vi "Ex 06 - B-Scan (DVR).vi"() -> ()   [LabVIEW 2015]
uses:
  <instrlib>/MicroPulse/Public/Data/Datatypes/MP - data formatting.ctl
  <instrlib>/MicroPulse/Public/Data/Datatypes/MP - amplitude reporting mode.ctl
  <instrlib>/MicroPulse/Public/Data/Datatypes/MP - averaging.ctl
  <instrlib>/MicroPulse/Public/Data/Datatypes/MP - transmit parameters.ctl
  <instrlib>/MicroPulse/Public/Data/Datatypes/MP - pulser voltage.ctl
  <instrlib>/MicroPulse/Public/Data/Datatypes/MP - pulse damping.ctl
  <instrlib>/MicroPulse/Public/Data/Datatypes/MP - test parameters.ctl
  <instrlib>/MicroPulse/Public/Data/Datatypes/MP - receive parameters.ctl
  <instrlib>/MicroPulse/Public/Data/Datatypes/MP - display gate.ctl
  <instrlib>/MicroPulse/Public/Data/Datatypes/MP - waveform type.ctl
  <instrlib>/MicroPulse/Public/Data/Datatypes/MP - analogue filter.ctl
  <instrlib>/MicroPulse/Public/Data/Datatypes/MP - frequency filter.ctl
  <instrlib>/MicroPulse/Public/Data/Datatypes/MP - digital filtering.ctl
  <instrlib>/MicroPulse/Public/Data/Datatypes/MP - high pass filter.ctl
  <instrlib>/MicroPulse/Public/Data/Datatypes/MP - low pass filter.ctl
  <instrlib>/MicroPulse/Public/Data/Datatypes/TCP config.ctl
  <instrlib>/MicroPulse/Public/Data/Datatypes/MP - multi-gate inspection.ctl
  <instrlib>/MicroPulse/Public/Data/Datatypes/MP - multigate inspection gate parameters.ctl
  <instrlib>/MicroPulse/Public/Data/Datatypes/MP - hysteresis level.ctl
  <instrlib>/MicroPulse/Public/Data/Datatypes/MP - multigate mode.ctl
  <instrlib>/MicroPulse/Public/Data/Datatypes/MP - echo gate parameters.ctl
  <instrlib>/MicroPulse/Public/Data/Datatypes/MP - echo gate mode.ctl
  <instrlib>/MicroPulse/Public/Data/Datatypes/MP - data output format.ctl
  <instrlib>/MicroPulse/Public/Data/Datatypes/MP - sample frequency.ctl
  <instrlib>/MicroPulse/Public/Data/Datatypes/MP - instrument type.ctl
  <instrlib>/MicroPulse/Public/Data/Datatypes/MP - fly scan range.ctl
  <instrlib>/MicroPulse/Public/Data/Datatypes/MP - inspection direction.ctl
  <instrlib>/MicroPulse/Public/Data/Datatypes/MP - encoder settings.ctl
  <instrlib>/MicroPulse/Public/Data/Datatypes/MP - encoder type.ctl
  <instrlib>/MicroPulse/Public/Data/Datatypes/MP - request system status.ctl
  <instrlib>/MicroPulse/Public/Data/Datatypes/MP - encoder mode.ctl
  <instrlib>/MicroPulse/Public/Data/Datatypes/MP - fly scan range (relative).ctl
  <instrlib>/MicroPulse/Public/Data/Datatypes/MP - inspection direction (relative).ctl
  <instrlib>/MicroPulse/Public/Data/Datatypes/MP - fly scan range (timed).ctl
  <instrlib>/MicroPulse/Public/Data/Datatypes/PNDT - colour map selector.ctl
  <instrlib>/MicroPulse/Examples/SubVIs/Main Program State - Enum.ctl
  <instrlib>/MicroPulse/Public/Data/Datatypes/MP - fly inspection tests.ctl
  <instrlib>/MicroPulse/Public/Helper VIs/Low Level/FGV - B-Scan Active - Action [Enum].ctl
  <vilib>/ErrorRing/Error Ring.xnode
  <instrlib>/MicroPulse/MicroPulse_Driver.lvlib
panel:
  in  "Centre Cursor":bool
  in  "Get Status":bool
  in  "Colour Map":T1
  out "B-Scan In Progress?":bool
  in  "Stop Test":bool
  out "B-Scan Chart":u16[][](graph)
  in  "Request System Status":T2 caption="[STS]"
  out "Current Position":dbl format="%#_6f mm"
  in  "Test Tab":T3(tab)
  in  "Data Formatting":T4={"Amplitude Mode"=enum."Peaks + Ascan for Multigate", "Averaging"=enum."None", "Coupling Level"=0} {"Coupling Level" max=4095 step=1}
  in  "Transmit Parameters":T7={"Pulse Voltage"=enum."50V", "Pulse Shape"={"Damping"=enum."660W", "Width"=250}} {"Pulse Shape"."Width" min=16 max=1010 step=50 format="%.0fns"}
  in  "Test Parameters":T10={"Test No."=1, "Tx Channel"=1, "Rx Channel"=1} {"Rx Channel" min=1 max=1024; "Tx Channel" min=1 max=1024}
  in  "Receive Parameters":T11={"Display Gate"={"Start"=0.0, "Length"=100.0}, "Delay"=0.0, "Waveform Type"=enum."Rectified Signal", "Gain"=50.0, "Analogue Filtering"={"Bandpass"=enum."No change", "Smoothing"=1}, "Digital Filtering"={"High Pass Filter"=enum."None", "Low Pass Filter"=enum."None"}} {"Delay" format="%#_g us"; "Display Gate"."Length" min=0.0 max=64000.0 step=1.0 format="%#_g us"; "Display Gate"."Start" min=0.0 max=64000.0 step=1.0 format="%#_g us"; "Analogue Filtering"."Smoothing" min=1 max=11 step=1; "Gain" min=-6.0 max=70.0 step=0.25 format="%.2fdB"}
  in  "Multi Gate Inspection":T19={"Gate 1"={"Start (us)"=15.0, "Length (us)"=10.0, "Threshold"=80, "Enabled?"=TRUE, "Max # Peaks"=8, "Hysteresis"=enum."6dB", "Mode"=enum."All Peaks In Gate", "Inverted?"=FALSE, "Colour "=16716306}, "Gate 2"={"Start (us)"=30.0, "Length (us)"=10.0, "Threshold"=50, "Enabled?"=TRUE, "Max # Peaks"=8, "Hysteresis"=enum."6dB", "Mode"=enum."All Peaks In Gate", "Inverted?"=FALSE, "Colour "=641024}, "Gate 3"={"Start (us)"=50.0, "Length (us)"=10.0, "Threshold"=30, "Enabled?"=TRUE, "Max # Peaks"=8, "Hysteresis"=enum."6dB", "Mode"=enum."All Peaks In Gate", "Inverted?"=FALSE, "Colour "=4532}, "Gate 4"={"Start (us)"=65.0, "Length (us)"=10.0, "Threshold"=10, "Enabled?"=TRUE, "Max # Peaks"=8, "Hysteresis"=enum."6dB", "Mode"=enum."All Peaks In Gate", "Inverted?"=FALSE, "Colour "=8978537}} {"Gate 4"."Max # Peaks" min=1 max=80 step=1; "Gate 4"."Threshold" min=10 step=10; "Gate 4"."Length (us)" min=0.0 max=96000.0 step=1.0; "Gate 4"."Start (us)" min=0.0 max=64000.0 step=1.0; "Gate 3"."Max # Peaks" min=1 max=80 step=1; "Gate 3"."Threshold" min=10 step=10; "Gate 3"."Length (us)" min=0.0 max=96000.0 step=1.0; "Gate 3"."Start (us)" min=0.0 max=64000.0 step=1.0; "Gate 2"."Max # Peaks" min=1 max=80 step=1; "Gate 2"."Threshold" min=10 step=10; "Gate 2"."Length (us)" min=0.0 max=96000.0 step=1.0; "Gate 2"."Start (us)" min=0.0 max=64000.0 step=1.0; "Gate 1"."Max # Peaks" min=1 max=80 step=1; "Gate 1"."Threshold" min=10 step=10; "Gate 1"."Length (us)" min=0.0 max=96000.0 step=1.0; "Gate 1"."Start (us)" min=0.0 max=64000.0 step=1.0}
  in  "Echo Gate Parameters":T23={"Start (us)"=15.0, "Length (us)"=20.0, "Threshold"=10, "Colour"=2731480} {"Threshold" min=10 max=4095 step=10; "Length (us)" min=0.0 max=96000.0 step=1.0; "Start (us)" min=0.0 max=64000.0 step=1.0}
  in  "Echo Gate Mode":T24
  in  "Encoder Reporting Mode":T25=enum."32-bit + LLC" caption="[ENCM]"
  in  "Set Position":bool
  in  "Position To Set":dbl caption="mm"
  in  "Encoder Settings":T26={"Encoder Type"=enum."Quadrature", "Counts/mm"=100, "Enable Termination?"=FALSE, "Multiplier"=2, "Backlash Period (s)"=10.0, "Encoder Filter"=0} {"Encoder Filter" max=255; "Backlash Period (s)" min=0.0005 max=10.0 step=0.0005; "Multiplier" min=1 max=100000; "Counts/mm" min=1 max=100000}
  in  "Axis No.":u8=1 min=1 max=4
  in  "Scan Choice":T28(tab)
  in  "FLZ Scan definition":T29={"Scan Start"=0.0, "Scan Length"=280.0, "Inspection Resolution"=0.5, "Direction"=enum."Forwards"} {"Inspection Resolution" format="%#_6f"; "Scan Start" format="%#_6f"; "Scan Length" format="%#_6f"}
  in  "Start FLZ Test":bool
  in  "FLR Scan definition":T31={"Scan Length"=0.0, "Inspection Resolution"=1.0, "Direction"=enum."Bidirectional"} {"Inspection Resolution" format="%#_6f"; "Scan Length" format="%#_6f"}
  in  "Start FLR Test":bool
  out "Scan Timer Enabled?":bool
  in  "Start Timed Test":bool
  in  "Timed Scan definition":T33={"Max Scan Length"=0, "Update Rate"=1000, "Direction"=enum."Forwards"} {"Update Rate" format="%#_6f"; "Max Scan Length" format="%#_6f"}
  out "Instrument Type":T34
  out "Sample Frequency out":T35 caption="Sample Frequency"
  out "Stop":bool
  in  "Sample Frequency":T35
  in  "PRF":u16=20000 caption="[PRF]" min=1 max=20000 step=100 format="%dHz"
  in  "Data Output Format":T36=enum."8-bit Mode" caption="[DOF]"
  in  "Gate No.":i32=1
  out "peak data":cluster{"Time":dbl[], "Level":u16[]} {"Time" format="%_6g"}
  out "A-Scan + Peaks":cluster{"timebase":dbl[], "data":u16[]}[](graph) caption="A-Scan + Peaks Test 1"
  in  "Acquire Single Scan":bool
  in  "Stop Acquisition":bool
  in  "Start Acquisition":bool
  out "Command List":string
  in  "QUIT":bool
  out "running average PRF":dbl format="%0.2f"
  out "live error out":errorcluster
  out "message count":i32
  out "System Messages":string
  in  "TCP config":T37={"Connection ID"=refnum, "IP address"="10.1.1.2", "host port"=1067, "OC timeout"=5000, "Read timeout"=2000, "Write timeout"=100} {"Write timeout" format="%dms"; "Read timeout" format="%dms"; "OC timeout" format="%dms"}
  # "Example 06 - B-Scans\n\nSet all controls to the required values\nbefore running the VI.\n\nWhile running, test parameters may NOT be  changed."
  # "Multiplier of 2 sets the inspection resolution to 1/2 of the base unit.\nBase unit is set by  \"Counts/mm\""
  # "Set Current Position"
  # "Set to zero for unlimited points. Requires manual stop."
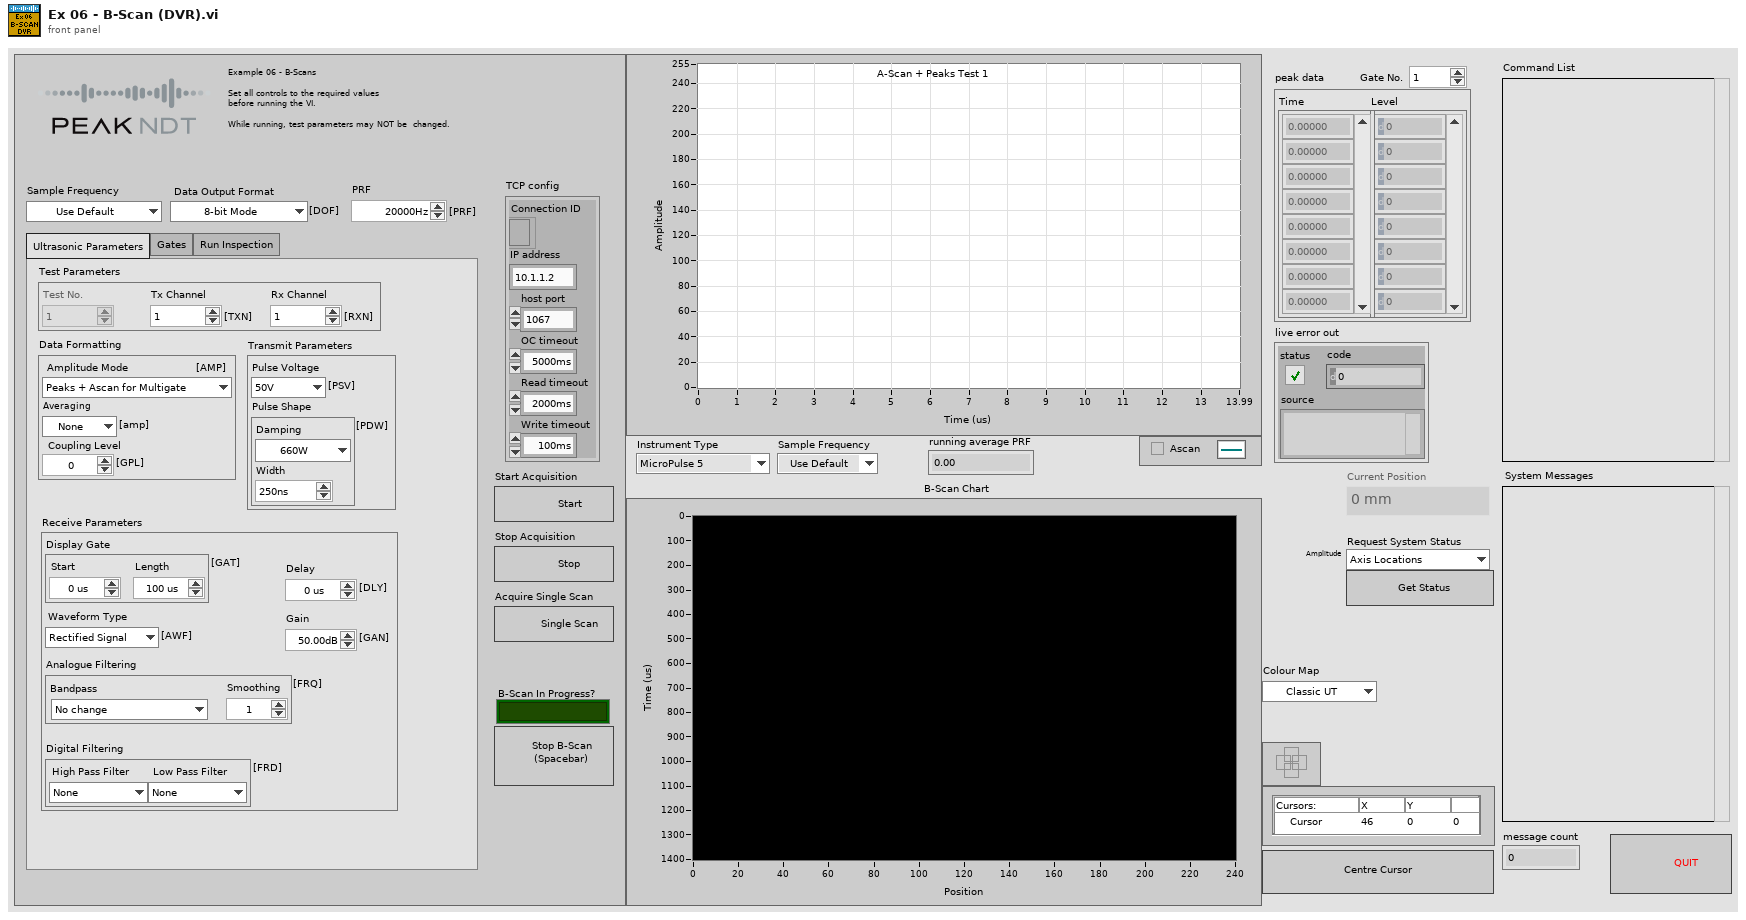
[diagram p1: front panel]
types:
  T1 = typedef "MicroPulse_Driver.lvlib/PNDT - colour map selector.ctl" = enum16{"Classic UT", "Ultrasonic", "Inverse Grey", "Grey Scale", "TOFD", "Fire", "Rainbow", "Ice", "Original"}
  T2 = typedef "MicroPulse_Driver.lvlib/MP - request system status.ctl" = enum16{"Axis Locations", "MPE settings", "BKL settings", "SPA settings", "I/O status", "RST elapsed time", "System Status", "Temperatures", "System Log", "Erase system Log", "RST message", "Master System Msg", "Slave System Msg"}
  T3 = enum32{"Ultrasonic Parameters", "Gates", "Run Inspection"}
  T4 = typedef "MicroPulse_Driver.lvlib/MP - data formatting.ctl" = cluster{"Amplitude Mode":T5, "Averaging":T6, "Coupling Level":u32}
  T5 = typedef "MicroPulse_Driver.lvlib/MP - amplitude reporting mode.ctl" = enum16{"1st Peak in gate", "Maximum Peak in gate", "All Peaks", "Ascan Data", "1st Threshold Crossing Peak", "Ascan + Peaks", "All Peaks for Multigate", "Peaks + Ascan for Multigate", "Peaks + P_Ascan for Multigate", "Full Matrix Capture"}
  T6 = typedef "MicroPulse_Driver.lvlib/MP - averaging.ctl" = enum16{"None", "2", "4", "8", "16", "32", "64", "128", "256"}
  T7 = typedef "MicroPulse_Driver.lvlib/MP - transmit parameters.ctl" = cluster{"Pulse Voltage":T8, "Pulse Shape":cluster{"Damping":T9, "Width":u32}}
  T8 = typedef "MicroPulse_Driver.lvlib/MP - pulser voltage.ctl" = enum16{"50V", "100V", "150V", "200V", "250V", "300V"}
  T9 = typedef "MicroPulse_Driver.lvlib/MP - pulse damping.ctl" = enum16{"660W", "458W", "220W", "149W", "102W", "82W", "63W", "51W"}
  T10 = typedef "MicroPulse_Driver.lvlib/MP - test parameters.ctl" = cluster{"Test No.":u32, "Tx Channel":u32, "Rx Channel":u32}
  T11 = typedef "MicroPulse_Driver.lvlib/MP - receive parameters.ctl" = cluster{"Display Gate":T12, "Delay":dbl, "Waveform Type":T13, "Gain":dbl, "Analogue Filtering":T14, "Digital Filtering":T16}
  T12 = typedef "MicroPulse_Driver.lvlib/MP - display gate.ctl" = cluster{"Start":dbl, "Length":dbl}
  T13 = typedef "MicroPulse_Driver.lvlib/MP - waveform type.ctl" = enum16{"Rectified Signal", "RF Signal", "+Half Wave", "-Half Wave"}
  T14 = typedef "MicroPulse_Driver.lvlib/MP - analogue filter.ctl" = cluster{"Bandpass":T15, "Smoothing":u16}
  T15 = typedef "MicroPulse_Driver.lvlib/MP - frequency filter.ctl" = enum16{"No change", "1MHz Bandpass", "2MHz Bandpass", "4MHz Bandpass", "5MHz Bandpass", "10MHz Bandpass", "2.5-18MHz Broadband", "0.75-12MHz  Broadband", "0.5MHz Bandpass", "5MHz 2nd Order TOFD", "10MHz 2nd Order TOFD", "3.0-25MHz Broadband", "3.0-30MHz Broadband"}
  T16 = typedef "MicroPulse_Driver.lvlib/MP - digital filtering.ctl" = cluster{"High Pass Filter":T17, "Low Pass Filter":T18}
  T17 = typedef "MicroPulse_Driver.lvlib/MP - high pass filter.ctl" = enum16{"None", "0.7MHz", "1.5MHz", "4.0MHz", "7.5MHz", "10.0MHz", "User Defined"}
  T18 = typedef "MicroPulse_Driver.lvlib/MP - low pass filter.ctl" = enum16{"None", "1.8MHz", "3.0MHz", "6.0MHz", "8.0MHz", "12.0MHz", "User Defined"}
  T19 = typedef "MicroPulse_Driver.lvlib/MP - multi-gate inspection.ctl" = cluster{"Gate 1":T20, "Gate 2":T20, "Gate 3":T20, "Gate 4":T20}
  T20 = typedef "MicroPulse_Driver.lvlib/MP - multigate inspection gate parameters.ctl" = cluster{"Start (us)":dbl, "Length (us)":dbl, "Threshold":u16, "Enabled?":bool, "Max # Peaks":u16, "Hysteresis":T21, "Mode":T22, "Inverted?":bool, "Colour ":u32}
  T21 = typedef "MicroPulse_Driver.lvlib/MP - hysteresis level.ctl" = enum16{"None", "3dB", "6dB", "9dB", "12dB"}
  T22 = typedef "MicroPulse_Driver.lvlib/MP - multigate mode.ctl" = enum16{"1st Peak in Gate", "Largest Peak In Gate", "All Peaks In Gate", "1st Threshold Crossing"}
  T23 = typedef "MicroPulse_Driver.lvlib/MP - echo gate parameters.ctl" = cluster{"Start (us)":dbl, "Length (us)":dbl, "Threshold":u16, "Colour":u32}
  T24 = typedef "MicroPulse_Driver.lvlib/MP - echo gate mode.ctl" = enum16{"Echo Trigger OFF", "Echo Gate Display Mode", "Echo Trigger ON", "Multi Gate or FMC Mode", "Reserved", "PA - Echo Trigger ON"}
  T25 = typedef "MicroPulse_Driver.lvlib/MP - encoder mode.ctl" = enum16{"24-bit + LCI", "32-bit + LCI", "32-bit + LLC", "24-bit + STS6", "32-bit + STS6", "32-bit + LLC+STS6"}
  T26 = typedef "MicroPulse_Driver.lvlib/MP - encoder settings.ctl" = cluster{"Encoder Type":T27, "Counts/mm":u32, "Enable Termination?":bool, "Multiplier":u32, "Backlash Period (s)":dbl, "Encoder Filter":u32}
  T27 = typedef "MicroPulse_Driver.lvlib/MP - encoder type.ctl" = enum16{"Quadrature", "Step/Direction"}
  T28 = enum32{"Absolute Scan [FLX+FLZ]", "Relative Scan [FLR] ", "Timed Scan"}
  T29 = typedef "MicroPulse_Driver.lvlib/MP - fly scan range.ctl" = cluster{"Scan Start":dbl, "Scan Length":dbl, "Inspection Resolution":dbl, "Direction":T30}
  T30 = typedef "MicroPulse_Driver.lvlib/MP - inspection direction.ctl" = enum16{"Forwards", "Backwards"}
  T31 = typedef "MicroPulse_Driver.lvlib/MP - fly scan range (relative).ctl" = cluster{"Scan Length":dbl, "Inspection Resolution":dbl, "Direction":T32}
  T32 = typedef "MicroPulse_Driver.lvlib/MP - inspection direction (relative).ctl" = enum16{"Forwards", "Backwards", "Bidirectional"}
  T33 = typedef "MicroPulse_Driver.lvlib/MP - fly scan range (timed).ctl" = cluster{"Max Scan Length":i32, "Update Rate":i32, "Direction":T30}
  T34 = typedef "MicroPulse_Driver.lvlib/MP - instrument type.ctl" = enum16{"MicroPulse 5", "LT1", "LT2", "LTPA", "MPLT", "MicroPulse 6", "PipeScanner", "<MicroPulse>", "Micropulse 4", "Simulated Data"}
  T35 = typedef "MicroPulse_Driver.lvlib/MP - sample frequency.ctl" = enum16{"Use Default", "200MHz (LT2 only)", "100MHz", "50MHz", "25MHz", "10MHz"}
  T36 = typedef "MicroPulse_Driver.lvlib/MP - data output format.ctl" = enum16{"", "8-bit Mode", "10-bit Mode", "12-bit Mode", "16-bit Mode", "8-bit Log Mode", "12-bit Packed Mode"}
  T37 = typedef "MicroPulse_Driver.lvlib/TCP config.ctl" = cluster{"Connection ID":refnum<k5>, "IP address":string, "host port":u16, "OC timeout":i32, "Read timeout":i32, "Write timeout":i32}
  T38 = typedef "Main Program State - Enum.ctl" = enum16{"Initialise", "Init HW", "Run", "Reset HW", "Shutdown"}
  T39 = typedef "MicroPulse_Driver.lvlib/FGV - B-Scan Active - Action [Enum].ctl" = enum16{"Read", "Read & Reset Start Flag", "Start B-Scan", "B-Scan Finished"}
  T40 = typedef "MicroPulse_Driver.lvlib/MP - fly inspection tests.ctl" = enum16{"Conventional Tests", "Conv >> PA Tests", "PA >> Conv Tests", "PA Tests", "Group Tests", "PA Sweep as per FDEF"}
  T41 = typedef "MicroPulse_Driver.lvlib/MP-Registry Data-Cluster.ctl" = cluster{"Instrument Type":T34, "Serial #":u64, "Sample Frequency":T35, "dt (us)":dbl, "DOF":T36, "Material Velocity":dbl, "Asynch Reads":T42, "NUM of Tests":u32, "System Details":T43, "Gates":T45[], "Encoders":T26[], "CMD LUT":variant, "Command List":string}
  T42 = typedef "MicroPulse_Driver.lvlib/MP - asynch read mode.ctl" = enum16{"Disabled", "Enabled"}
  T43 = typedef "MicroPulse_Driver.lvlib/MP - general system status.ctl" = cluster{"System Type":T34, "Serial No.":u64, "Channels":cluster{"Conv":u8, "PA":u16, "Extra":u32}, "Sample Frequency":cluster{"Default":u8, "Actual":u8}, "Software Versions":string, "Data Output Format":cluster{"Default":T36, "Actual":T36}, "Temperatures":cluster{"System":u8, "Processor":u8, "Slave Sys":u8, "Slave Proc":u8}, "Tx Buffer Size":u32, "System Error":string, "No. of Cards":u8, "DAC Gain":i16, "Uptimes":cluster{"since Power":u32, "since RSTS":u32, "since SRST":u32}, "Voltages":cluster{"Nominal":dbl, "Measured":dbl, "Difference":dbl}[], "Interface Cards":T44[]}
  T44 = typedef "MicroPulse_Driver.lvlib/MP - interface card status.ctl" = cluster{"Status":u8, "Map":u8, "Board - T":u8, "FPGA - T":u8, "PAIF Status":string, "Version":string}
  T45 = typedef "MicroPulse_Driver.lvlib/MP - Registry Gates.ctl" = cluster{"Display Gate":T12, "ETM Mode":T24, "Echo Gate":T23, "Insp Gates":T20[]}
  T46 = typedef "LVPointDoubleTypeDef.ctl" = cluster{"Cursor X":dbl, "Cursor Y":dbl}
  T47 = typedef "LVBoundsTypeDef.ctl" = cluster{"Width":u32, "Height":u32}
  T48 = typedef "MicroPulse_Driver.lvlib/MP - scan data info.ctl" = cluster{"Message Header":u16, "Error Message":u16, "Test No.":u32, "Channel No.":u8, "Sweep No.":u32, "Gate No.":u32, "DOF":T36, "retain data":T49, "scan data":u16[], "scan length":i32, "scan index":i32, "peak data":cluster{"timebase":u16[], "data":u16[]}, "#peaks":i32, "PRF":dbl, "IP":cluster{"Axis No.":u8, "Location":u32, "MIP location":u32, "MIP?":bool}, "echo range":u16, "ETG":bool, "CAL 0 complete":bool, "Axis Positions":T50}
  T49 = typedef "MicroPulse_Driver.lvlib/MP - retain scan.ctl" = enum16{"None", "Ascan", "Peaks"}
  T50 = typedef "MicroPulse_Driver.lvlib/MP - axis positions (LLC).ctl" = cluster{"Axis 1":u32, "Axis 2":u32, "Axis 3":u32, "Axis 4":u32, "Status":u8}
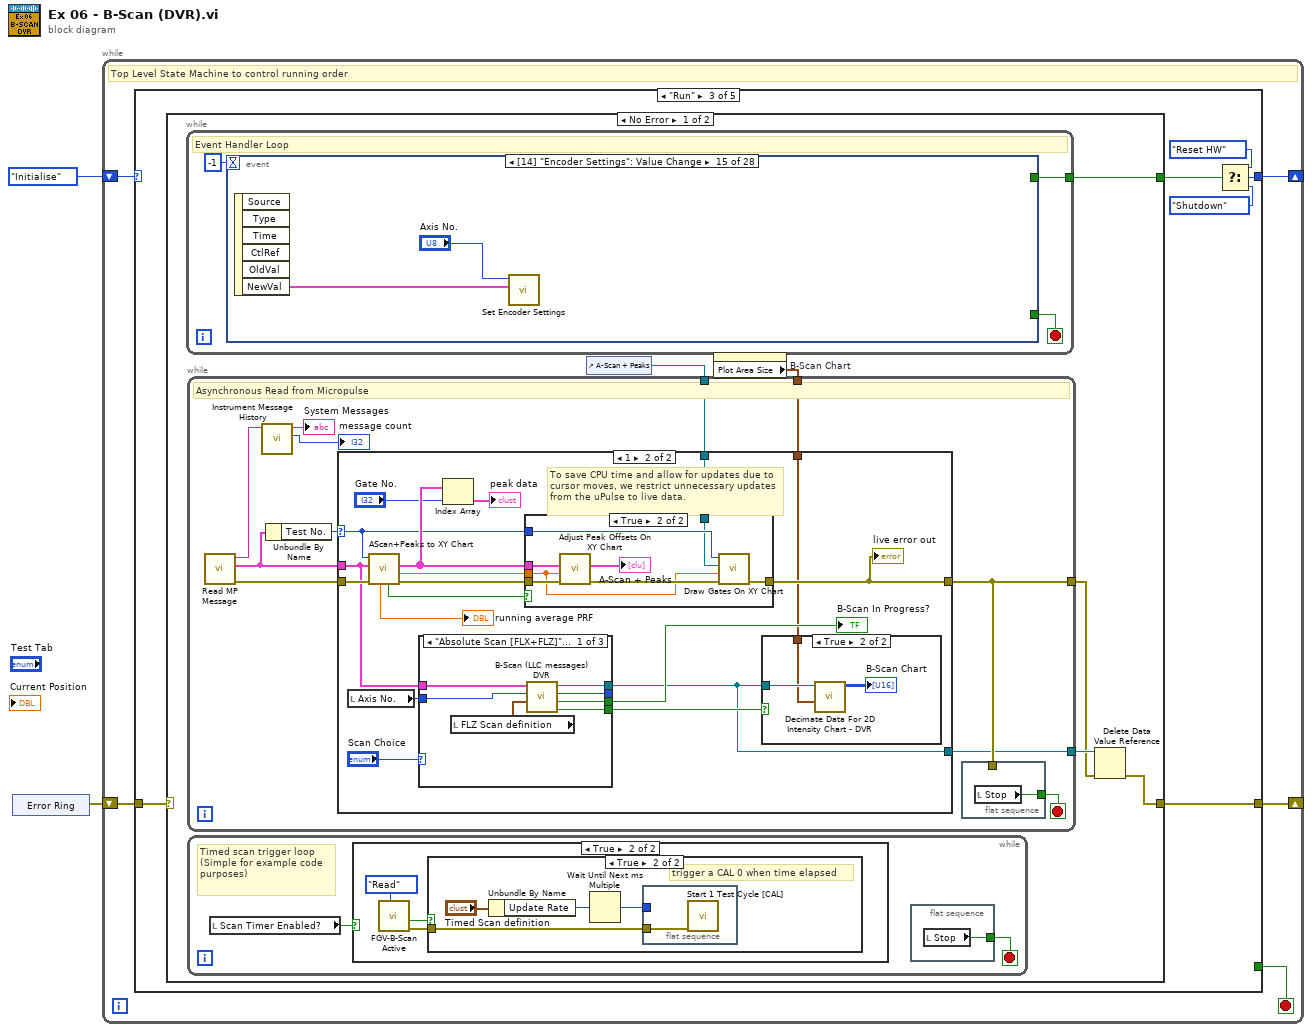
[diagram p0: block diagram]
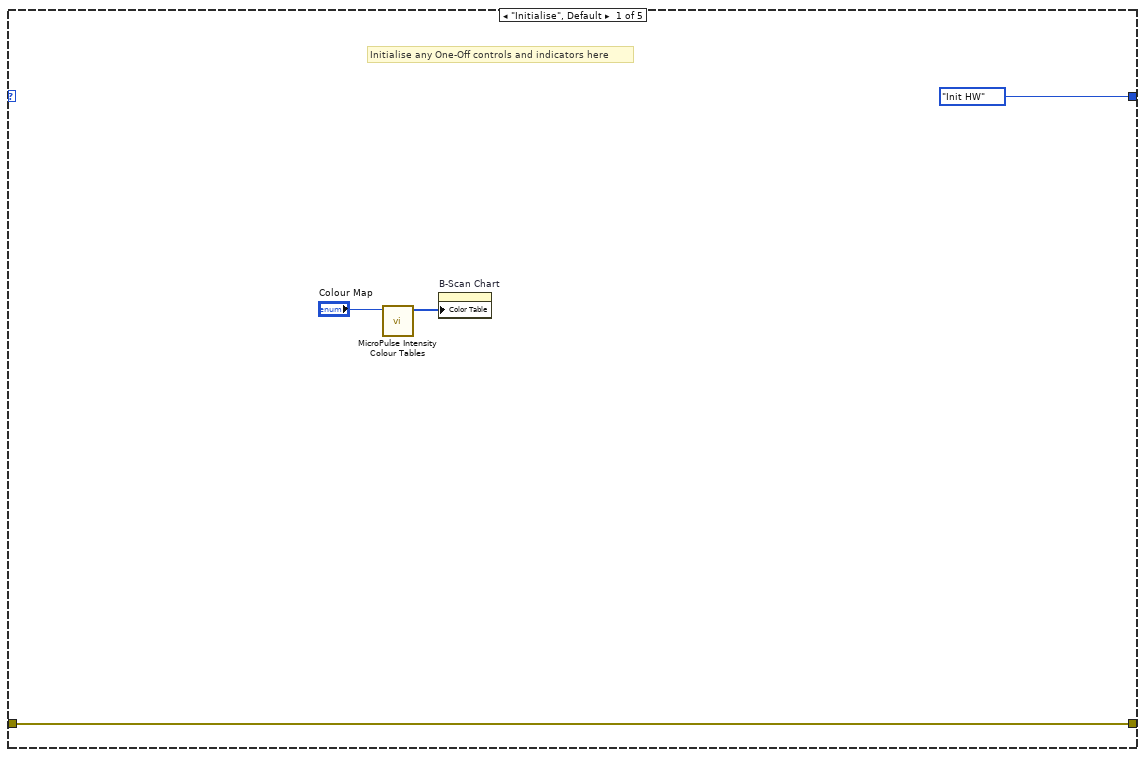
[diagram p2: hidden frame]
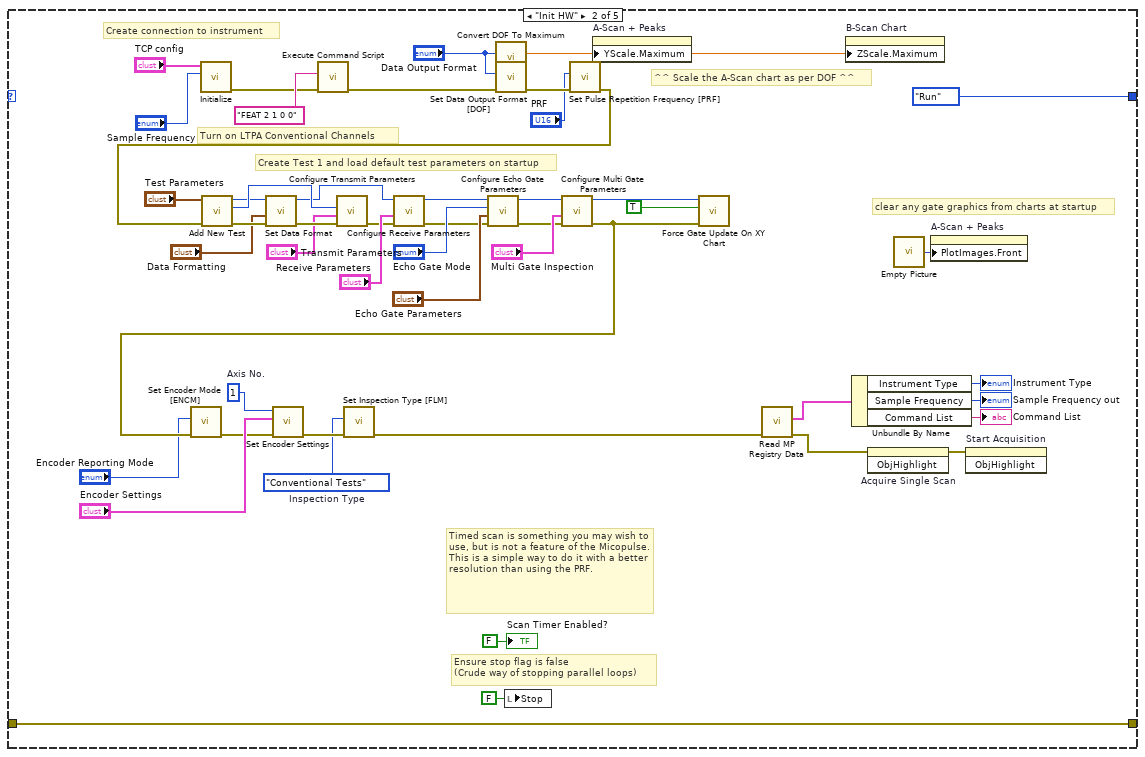
[diagram p3: hidden frame]
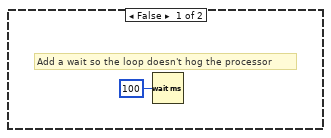
[diagram p4: hidden frame]
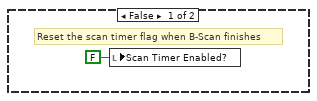
[diagram p5: hidden frame]
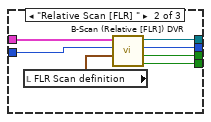
[diagram p9: hidden frame]
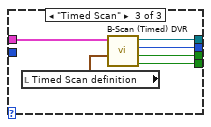
[diagram p10: hidden frame]
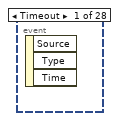
[diagram p11: hidden frame]
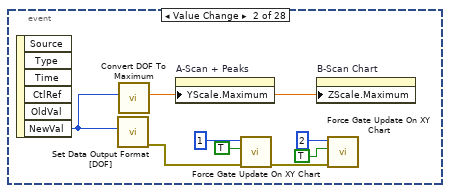
[diagram p12: hidden frame]
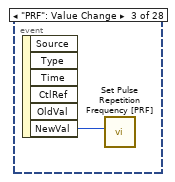
[diagram p13: hidden frame]
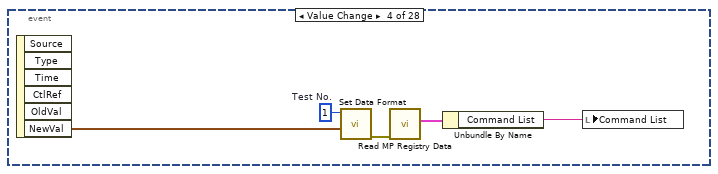
[diagram p14: hidden frame]
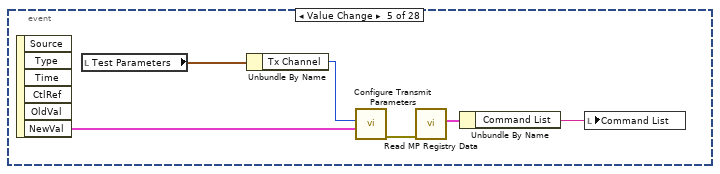
[diagram p15: hidden frame]
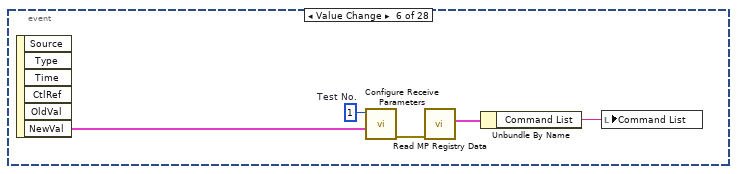
[diagram p16: hidden frame]
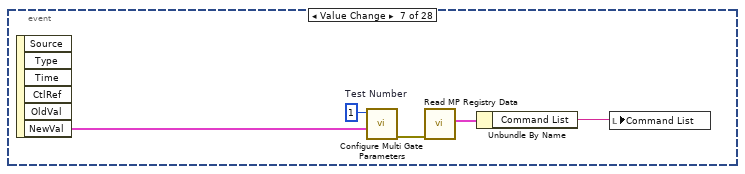
[diagram p17: hidden frame]
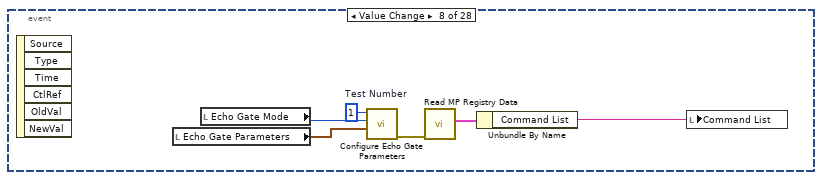
[diagram p18: hidden frame]
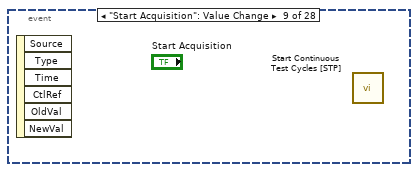
[diagram p19: hidden frame]
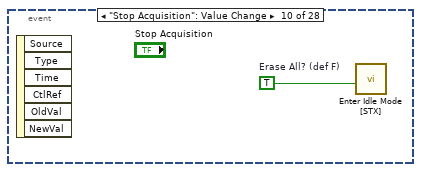
[diagram p20: hidden frame]
diagram:
  n1 = xnode "Error Ring"() -> ("error out"=w2:errorcluster)
  n2 = while {
    shift-right: [w4] -> _
    shift-left: Main_Program_State_-_Enum."Initialise" -> [w7]
    shift-right: [w5] -> _
    shift-left: w2 -> [w6]
    stop <- w3 stop-if-true
    # "Top Level State Machine to control running order"
    n3 = case shown="\"Run\"" w7 {
      tunnel: w6 -> [w10 w37 w65 w256 w261]
      tunnel: [w10 w37 w64 w255 w261] -> w5
      tunnel: [Main_Program_State_-_Enum."Init HW" Main_Program_State_-_Enum."Run" w60 Main_Program_State_-_Enum."Init HW" Main_Program_State_-_Enum."Initialise"] -> w4
      tunnel: [_ _ _ _ TRUE] -> w3
      frame "Initialise", Default {
        # "Initialise any One-Off controls and indicators here"
        n4 = call <instrlib>:"MicroPulse Intensity Colour Tables.vi"("Colour Map Type"="Colour Map") -> ("Colour Table"=w8:u32[])  [unwired: 10 in]
        n5 = property on="B-Scan Chart" class="IntGraph (strict)"("Color Table"=w8) -> ()  [unwired: 2 in, 2 out]
      }
      frame "Init HW" {
        w17 = MP_-_fly_inspection_tests."Conventional Tests"  # Inspection Type
        w20 = u8 1  # Axis No.
        # "Turn on LTPA Conventional Channels"
        # "Timed scan is something you may wish to use, but is not a feature of the Micopulse.\nThis is a simple way to do it with a better resolution than using the PRF."
        # "^^ Scale the A-Scan chart as per DOF ^^"
        # "Ensure stop flag is false\n(Crude way of stopping parallel loops)"
        # "Create connection to instrument"
        # "clear any gate graphics from charts at startup"
        # "Create Test 1 and load default test parameters on startup"
        n6 = call <instrlib>:"Initialize.vi"("Sample Frequency"="Sample Frequency", "TCP config"="TCP config") -> ("error out"=w13:errorcluster)  [unwired: 8 in, 1 out]
        n7 = call <instrlib>:"Execute Command Script.vi"("error in (no error)"=w13, "String in"="FEAT 2 1 0 0") -> ("error out"=w12:errorcluster)  [unwired: 7 in, 2 out]
        n8 = call <instrlib>:"Convert DOF To Maximum.vi"("Data Output Format"="Data Output Format") -> ("Data Maximum"=w16:dbl)  [unwired: 10 in]
        n9 = call <instrlib>:"Set Data Output Format [DOF].vi"("error in (no error)"=w12, "Mode"="Data Output Format") -> ("error out"=w30:errorcluster)  [unwired: 8 in, 1 out]
        n10 = local write "Stop"(FALSE ("stop")) -> ()
        n11 = call <instrlib>:"Set Pulse Repetition Frequency [PRF].vi"("error in (no error)"=w30, "Frequency (Hz)"="PRF") -> ("error out"=w28:errorcluster)  [unwired: 8 in, 1 out]
        n12 = call <instrlib>:"Add New Test.vi"("error in (no error)"=w28, "Test Parameters"="Test Parameters") -> ("error out"=w52:errorcluster, "Tx Channel out"=w51:u32, "Test No. out"=w47:u32)  [unwired: 6 in, 1 out]
        n13 = call <instrlib>:"Set Data Format.vi"("error in (no error)"=w52, "Data Formatting"="Data Formatting", "Test No."=w47) -> ("error out"=w42:errorcluster, "Test No. out"=w49:u32)  [unwired: 6 in, 1 out]
        n14 = call <instrlib>:"Configure Transmit Parameters.vi"("error in (no error)"=w42, "Transmit Parameters"="Transmit Parameters", "Tx Channel"=w51) -> ("error out"=w41:errorcluster)  [unwired: 7 in, 1 out]
        n15 = call <instrlib>:"Configure Receive Parameters.vi"("error in (no error)"=w41, "Receive Parameters"="Receive Parameters", "Test No."=w49) -> ("error out"=w43:errorcluster, "Test No. out"=w48:u32)  [unwired: 6 in, 1 out]
        n16 = call <instrlib>:"Configure Echo Gate Parameters.vi"("error in (no error)"=w43, "Echo Gate Parameters"="Echo Gate Parameters", "Echo Trigger Mode"="Echo Gate Mode", "Test Number"=w48) -> ("error out"=w45:errorcluster, "Test Number Out"=w50:u32)  [unwired: 5 in, 1 out]
        n17 = call <instrlib>:"Configure Multi Gate Parameters.vi"("error in (no error)"=w45, "Multi Gate Inspection"="Multi Gate Inspection", "Test Number"=w50) -> ("error out"=w24:errorcluster, "Test Number out"=w35:u32)  [unwired: 6 in, 1 out]
        n18 = call <instrlib>:"Set Encoder Mode [ENCM].vi"("error in (no error)"=w24, "Encoder Mode"="Encoder Reporting Mode") -> ("error out"=w21:errorcluster)  [unwired: 8 in, 1 out]
        n19 = call <instrlib>:"Set Encoder Settings.vi"("error in (no error)"=w21, "Encoder Settings"="Encoder Settings", "Axis No."=w20) -> ("error out"=w19:errorcluster)  [unwired: 8 in]
        n20 = call <instrlib>:"Set Inspection Type [FLM].vi"("error in (no error)"=w19, "Inspection Type"=w17) -> ("error out"=w18:errorcluster)  [unwired: 8 in, 1 out]
        n21 = property on="A-Scan + Peaks" class="XYGraph (strict)"("YScale.Maximum"=w16) -> ()  [unwired: 2 in, 2 out]
        n22 = call <instrlib>:"Force Gate Update On XY Chart.vi"("error in (no error)"=w24, "Set?"=TRUE, "Test No."=w35) -> ()  [unwired: 6 in, 3 out]
        n23 = call <instrlib>:"Read MP Registry Data.vi"("error in (no error)"=w18) -> ("error out"=w58:errorcluster, "Micropulse Data"=w56:T41)  [unwired: 7 in, 2 out]
        n24 = property on="B-Scan Chart" class="IntGraph (strict)"("ZScale.Maximum"=w16) -> ()  [unwired: 2 in, 2 out]
        n25 = Unbundle By Name(w56) -> ("Instrument Type"=→"Instrument Type":T34, "Sample Frequency"=→"Sample Frequency out":T35, "Command List"=→"Command List":string)
        n26 = invoke on="Acquire Single Scan" class="Bool" method="ObjHighlight"(error in=w58) -> (error out=w59:errorcluster)  [unwired: 2 in, 2 out]
        n27 = call "Empty Picture"() -> ("empty picture"=w36:picture)
        n28 = property on="A-Scan + Peaks" class="XYGraph (strict)"("PlotImages.Front"=w36) -> ()  [unwired: 2 in, 2 out]
        n29 = invoke on="Start Acquisition" class="Bool" method="ObjHighlight"(error in=w59) -> ()  [unwired: 2 in, 3 out]
        "Scan Timer Enabled?" <- FALSE ("Scan Timer Enabled?")
      }
      frame "Run" {
        n30 = case shown="No Error" w65 {
          selector: w65 -> [_ w254]
          tunnel: [w67 w254] -> w64
          tunnel: [w70 FALSE] -> w61
          frame No Error {
            n31 = while {
              tunnel: [w149] -> w70
              stop <- w150 stop-if-true
              # "Event Handler Loop"
              n32 = event shown="[14] \"Encoder Settings\": Value Change" {
                selector: _ -> [_ _ _ _ _ _ _ _ _ _ _ _ _ _ _ _ _ _ _ _ _ _ _ _ _ _ _ _]
                dyn-events: _ -> [_ _ _ _ _ _ _ _ _ _ _ _ _ _ _ _ _ _ _ _ _ _ _ _ _ _ _ _]
                timeout: -1 -> [_ _ _ _ _ _ _ _ _ _ _ _ _ _ _ _ _ _ _ _ _ _ _ _ _ _ _ _]
                tunnel: [_ _ _ _ _ _ _ _ _ _ _ _ w190 _ _ _ _ _ _ _ _ _ _ _ _ _ _ TRUE ("stop")] -> w150
                tunnel: [_ _ _ _ _ _ _ _ _ _ _ _ TRUE _ _ _ _ _ _ _ _ _ _ _ _ _ FALSE _] -> w149
                event Timeout {
                  n33 = event-data() -> ()  [unwired: 1 in, 3 out]
                }
                event Value Change {
                  n34 = event-data() -> ("NewVal"=w152:T36)  [unwired: 1 in, 5 out]
                  n35 = call <instrlib>:"Set Data Output Format [DOF].vi"("Mode"=w152) -> ("error out"=w154:errorcluster)  [unwired: 9 in, 1 out]
                  n36 = call <instrlib>:"Convert DOF To Maximum.vi"("Data Output Format"=w152) -> ("Data Maximum"=w151:dbl)  [unwired: 10 in]
                  n37 = property on="A-Scan + Peaks" class="XYGraph (strict)"("YScale.Maximum"=w151) -> ()  [unwired: 2 in, 2 out]
                  n38 = call <instrlib>:"Force Gate Update On XY Chart.vi"("error in (no error)"=w154, "Set?"=TRUE, "Test No."=u32 1) -> ("error out"=w153:errorcluster)  [unwired: 6 in, 2 out]
                  n39 = property on="B-Scan Chart" class="IntGraph (strict)"("ZScale.Maximum"=w151) -> ()  [unwired: 2 in, 2 out]
                  n40 = call <instrlib>:"Force Gate Update On XY Chart.vi"("error in (no error)"=w153, "Set?"=TRUE, "Test No."=u32 2) -> ()  [unwired: 6 in, 3 out]
                }
                event "PRF": Value Change {
                  n41 = event-data() -> ("NewVal"=w159:u16)  [unwired: 1 in, 5 out]
                  n42 = call <instrlib>:"Set Pulse Repetition Frequency [PRF].vi"("Frequency (Hz)"=w159) -> ()  [unwired: 9 in, 2 out]
                }
                event Value Change {
                  w161 = u32 1  # Test No.
                  n43 = event-data() -> ("NewVal"=w160:T4)  [unwired: 1 in, 5 out]
                  n44 = call <instrlib>:"Set Data Format.vi"("Data Formatting"=w160, "Test No."=w161) -> ("error out"=w164:errorcluster)  [unwired: 7 in, 2 out]
                  n45 = call <instrlib>:"Read MP Registry Data.vi"("error in (no error)"=w164) -> ("Micropulse Data"=w163:T41)  [unwired: 7 in, 3 out]
                  n46 = Unbundle By Name(w163) -> ("Command List"=w162:string)
                  n47 = local write "Command List"(w162) -> ()
                }
                event Value Change {
                  n48 = event-data() -> ("NewVal"=w169:T7)  [unwired: 1 in, 5 out]
                  n49 = local read "Test Parameters"() -> (w170:T10)
                  n50 = Unbundle By Name(w170) -> ("Tx Channel"=w168:u32)
                  n51 = call <instrlib>:"Configure Transmit Parameters.vi"("Transmit Parameters"=w169, "Tx Channel"=w168) -> ("error out"=w166:errorcluster)  [unwired: 8 in, 1 out]
                  n52 = call <instrlib>:"Read MP Registry Data.vi"("error in (no error)"=w166) -> ("Micropulse Data"=w167:T41)  [unwired: 7 in, 3 out]
                  n53 = Unbundle By Name(w167) -> ("Command List"=w165:string)
                  n54 = local write "Command List"(w165) -> ()
                }
                event Value Change {
                  w171 = u32 1  # Test No.
                  n55 = event-data() -> ("NewVal"=w175:T11)  [unwired: 1 in, 5 out]
                  n56 = call <instrlib>:"Configure Receive Parameters.vi"("Receive Parameters"=w175, "Test No."=w171) -> ("error out"=w174:errorcluster)  [unwired: 7 in, 2 out]
                  n57 = call <instrlib>:"Read MP Registry Data.vi"("error in (no error)"=w174) -> ("Micropulse Data"=w172:T41)  [unwired: 7 in, 3 out]
                  n58 = Unbundle By Name(w172) -> ("Command List"=w173:string)
                  n59 = local write "Command List"(w173) -> ()
                }
                event Value Change {
                  w176 = u32 1  # Test Number
                  n60 = event-data() -> ("NewVal"=w180:T19)  [unwired: 1 in, 5 out]
                  n61 = call <instrlib>:"Configure Multi Gate Parameters.vi"("Multi Gate Inspection"=w180, "Test Number"=w176) -> ("error out"=w179:errorcluster)  [unwired: 7 in, 2 out]
                  n62 = call <instrlib>:"Read MP Registry Data.vi"("error in (no error)"=w179) -> ("Micropulse Data"=w178:T41)  [unwired: 7 in, 3 out]
                  n63 = Unbundle By Name(w178) -> ("Command List"=w177:string)
                  n64 = local write "Command List"(w177) -> ()
                }
                event Value Change {
                  w181 = u32 1  # Test Number
                  n65 = event-data() -> ()  [unwired: 1 in, 6 out]
                  n66 = local read "Echo Gate Parameters"() -> (w184:T23)
                  n67 = local read "Echo Gate Mode"() -> (w185:T24)
                  n68 = call <instrlib>:"Configure Echo Gate Parameters.vi"("Echo Gate Parameters"=w184, "Echo Trigger Mode"=w185, "Test Number"=w181) -> ("error out"=w186:errorcluster)  [unwired: 6 in, 2 out]
                  n69 = call <instrlib>:"Read MP Registry Data.vi"("error in (no error)"=w186) -> ("Micropulse Data"=w183:T41)  [unwired: 7 in, 3 out]
                  n70 = Unbundle By Name(w183) -> ("Command List"=w182:string)
                  n71 = local write "Command List"(w182) -> ()
                }
                event "Start Acquisition": Value Change {
                  n72 = event-data() -> ()  [unwired: 1 in, 6 out]
                  n73 = call <instrlib>:"Start Continuous Test Cycles [STP].vi"() -> ()  [unwired: 10 in, 2 out]
                }
                event "Stop Acquisition": Value Change {
                  w187 = TRUE  # Erase All? (def F)
                  n74 = event-data() -> ()  [unwired: 1 in, 6 out]
                  n75 = call <instrlib>:"Enter Idle Mode [STX].vi"("Erase All? (def T)"=w187) -> ()  [unwired: 9 in, 2 out]
                }
                event "Acquire Single Scan": Value Change {
                  n76 = event-data() -> ()  [unwired: 1 in, 6 out]
                  n77 = call <instrlib>:"Start 1 Test Cycle [CAL].vi"() -> ()  [unwired: 10 in, 2 out]
                }
                event "A-Scan + Peaks": Scale Range Change {
                  n78 = event-data() -> ()  [unwired: 1 in, 8 out]
                  n79 = call <instrlib>:"Force Gate Update On XY Chart.vi"("Set?"=TRUE, "Test No."=u32 1) -> ()  [unwired: 7 in, 3 out]
                }
                event Value Change {
                  w190 = TRUE
                  # "Stop all activity and reset the hardware to change the sampling frequency"
                  n80 = event-data() -> ()  [unwired: 1 in, 6 out]
                  n81 = local write "Stop"(w190) -> ()
                }
                event Value Change {
                  n82 = event-data() -> ("NewVal"=w192:T25)  [unwired: 1 in, 5 out]
                  n83 = call <instrlib>:"Set Encoder Mode [ENCM].vi"("Encoder Mode"=w192) -> ()  [unwired: 9 in, 2 out]
                }
                event Value Change {
                  n84 = event-data() -> ("NewVal"=w194:T26)  [unwired: 1 in, 5 out]
                  n85 = call <instrlib>:"Set Encoder Settings.vi"("Encoder Settings"=w194, "Axis No."="Axis No.") -> ()  [unwired: 9 in, 1 out]
                }
                event "Set Position": Value Change {
                  w195 = u8 1  # Axis No.
                  n86 = event-data() -> ()  [unwired: 1 in, 6 out]
                  n87 = call <instrlib>:"Set Encoder Position [LCP].vi"("Position (mm)"="Position To Set", "Axis No."=w195) -> ()  [unwired: 8 in, 2 out]
                }
                event Value Change {
                  n88 = event-data() -> ()  [unwired: 1 in, 6 out]
                }
                event Value Change {
                  n89 = event-data() -> ("NewVal"=w198:T1)  [unwired: 1 in, 5 out]
                  n90 = call <instrlib>:"MicroPulse Intensity Colour Tables.vi"("Colour Map Type"=w198) -> ("Colour Table"=w197:u32[])  [unwired: 10 in]
                  n91 = property on="B-Scan Chart" class="IntGraph (strict)"("Color Table"=w197) -> ()  [unwired: 2 in, 2 out]
                }
                event "Get Status": Value Change {
                  n92 = event-data() -> ()  [unwired: 1 in, 6 out]
                  n93 = call <instrlib>:"Get Status Info [STS].vi"("Request System Status"="Request System Status") -> ()  [unwired: 9 in, 2 out]
                }
                event "Start FLZ Test": Value Change {
                  w205 = u8 1  # Axis No.
                  # "Stop any acquisition that's going on"
                  n94 = event-data() -> ()  [unwired: 1 in, 6 out]
                  n95 = call <instrlib>:"Enter Idle Mode [STX].vi"() -> ("error out"=w207:errorcluster)  [unwired: 10 in, 1 out]
                  n96 = call <instrlib>:"Start Scan (Start to End).vi"("error in (no error)"=w207, "Scan definition"="FLZ Scan definition", "Axis No."=w205) -> ("error out"=w204:errorcluster)  [unwired: 7 in, 1 out]
                  n97 = call <instrlib>:"FGV-B-Scan Active.vi"("Action"=FGV_-_B-Scan_Active_-_Action_[Enum]."Start B-Scan", "error in (no error)"=w204) -> ("error out"=w201:errorcluster)  [unwired: 7 in, 2 out]
                  n98 = call <instrlib>:"Read MP Registry Data.vi"("error in (no error)"=w201) -> ("Micropulse Data"=w203:T41)  [unwired: 7 in, 3 out]
                  n99 = Unbundle By Name(w203) -> ("Command List"=w202:string)
                  n100 = local write "Command List"(w202) -> ()
                }
                event "Start FLR Test": Value Change {
                  w209 = u8 1  # Axis No.
                  # "Stop any acquisition that's going on"
                  n101 = event-data() -> ()  [unwired: 1 in, 6 out]
                  n102 = call <instrlib>:"Enter Idle Mode [STX].vi"() -> ("error out"=w211:errorcluster)  [unwired: 10 in, 1 out]
                  n103 = call <instrlib>:"Start Scan (Relative [FLR]).vi"("error in (no error)"=w211, "Scan definition"="FLR Scan definition", "Axis No."=w209) -> ("error out"=w210:errorcluster)  [unwired: 7 in, 1 out]
                  n104 = call <instrlib>:"FGV-B-Scan Active.vi"("Action"=FGV_-_B-Scan_Active_-_Action_[Enum]."Start B-Scan", "error in (no error)"=w210) -> ("error out"=w213:errorcluster)  [unwired: 7 in, 2 out]
                  n105 = call <instrlib>:"Read MP Registry Data.vi"("error in (no error)"=w213) -> ("Micropulse Data"=w215:T41)  [unwired: 7 in, 3 out]
                  n106 = Unbundle By Name(w215) -> ("Command List"=w214:string)
                  n107 = local write "Command List"(w214) -> ()
                }
                event "Start Timed Test": Value Change {
                  # "use property node so we can sequence starting\nthe B-Scan acitve flags and then enabling the timer"
                  # "Stop any acquisition that's going on"
                  n108 = event-data() -> ()  [unwired: 1 in, 6 out]
                  n109 = call <instrlib>:"Enter Idle Mode [STX].vi"() -> ("error out"=w218:errorcluster)  [unwired: 10 in, 1 out]
                  n110 = call <instrlib>:"FGV-B-Scan Active.vi"("Action"=FGV_-_B-Scan_Active_-_Action_[Enum]."Start B-Scan", "error in (no error)"=w218) -> ("error out"=w217:errorcluster)  [unwired: 7 in, 2 out]
                  n111 = property on="Scan Timer Enabled?" class="Bool (strict)"(error in=w217, "Value"=TRUE ("Scan Timer Enabled?")) -> ()  [unwired: 1 in, 2 out]
                }
                event Key Down {
                  n112 = event-data() -> ("Char"=w220:i16)  [unwired: 1 in, 7 out]
                  n113 = case shown="32" w220 {
                    frame 0, Default {
                    }
                    frame 32 {
                      # "Space bar - Stops all scan activity - returns micropulse to idle mode"
                      n114 = call <instrlib>:"FGV-B-Scan Active.vi"() -> ("B-Scan In Progress?"=w221:bool)  [unwired: 9 in, 2 out]
                      n115 = case shown="True" w221 {
                        frame False {
                        }
                        frame True {
                          n116 = call <instrlib>:"Enter Idle Mode [STX].vi"() -> ("error out"=w222:errorcluster)  [unwired: 10 in, 1 out]
                          n117 = call <instrlib>:"FGV-B-Scan Active.vi"("Action"=FGV_-_B-Scan_Active_-_Action_[Enum]."B-Scan Finished", "error in (no error)"=w222) -> ()  [unwired: 7 in, 3 out]
                        }
                      }
                    }
                  }
                }
                event "Stop Test": Value Change {
                  # "Stops all scan activity - returns micropulse to idle mode\nHitting the Spacebar also does this."
                  n118 = event-data() -> ()  [unwired: 1 in, 5 out]
                  n119 = call <instrlib>:"FGV-B-Scan Active.vi"() -> ("B-Scan In Progress?"=w224:bool)  [unwired: 9 in, 2 out]
                  n120 = case shown="True" w224 {
                    frame False {
                    }
                    frame True {
                      n121 = call <instrlib>:"Enter Idle Mode [STX].vi"() -> ("error out"=w225:errorcluster)  [unwired: 10 in, 1 out]
                      n122 = call <instrlib>:"FGV-B-Scan Active.vi"("Action"=FGV_-_B-Scan_Active_-_Action_[Enum]."B-Scan Finished", "error in (no error)"=w225) -> ()  [unwired: 7 in, 3 out]
                    }
                  }
                }
                event "Centre Cursor": Value Change {
                  n123 = event-data() -> ()  [unwired: 1 in, 6 out]
                  n124 = property on="B-Scan Chart" class="IntGraph (strict)"() -> ("XScale.Maximum"=w232:dbl, "XScale.Minimum"=w228:dbl)  [unwired: 2 in, 2 out]
                  n125 = Subtract(x=w232, y=w228) -> (x-y=w231:dbl)
                  n126 = Divide(x=w231, y=2.0) -> (x/y=w229:dbl)
                  n127 = Add(x=w229, y=w228) -> (x+y=w227:dbl)
                  n128 = property on="B-Scan Chart" class="IntGraph (strict)"("Cursor.Cursor X"=w227) -> ()  [unwired: 2 in, 2 out]
                }
                event "B-Scan Chart": Cursor Move {
                  n129 = event-data() -> ()  [unwired: 1 in, 8 out]
                  n130 = property on="B-Scan Chart" class="IntGraph (strict)"() -> ("Cursor.Cursor Position"=w233:T46, "Value"=w241:u16[][])  [unwired: 2 in, 2 out]
                  n131 = Unbundle By Name(w233) -> ("Cursor X"=w240:dbl)
                  n132 = property on="A-Scan + Peaks" class="XYGraph (strict)"() -> ("XScale.Multiplier"=w239:dbl, "XScale.Offset"=w238:dbl)  [unwired: 2 in, 2 out]
                  n133 = Index Array(array=w241, index (row)=w240) -> (element=w236:u16[])  [unwired: 1 in]
                  n134 = for {
                    tunnel: w236 -> [_] mode=indexing
                    tunnel: w239 -> [w246]
                    tunnel: w238 -> [w243]
                    tunnel: [w242] -> w237 mode=indexing
                    i -> [w245]
                    n135 = Multiply(x=w246, y=w245) -> (x*y=w244:dbl)
                    n136 = Subtract(x=w244, y=w243) -> (x-y=w242:dbl)
                  }
                  n137 = Bundle(w237, "Value"=w236) -> (w235:cluster{dbl[], "Value":u16[]})  [unwired: 1 in]
                  n138 = Build Array(w235) -> (w234:cluster{dbl[], "Value":u16[]}[])
                  n139 = local write "A-Scan + Peaks"(w234) -> ()
                }
                event Panel Close? {
                  n140 = event-data() -> ()  [unwired: 1 in, 4 out]
                  n141 = event-data("Discard?"=TRUE) -> ()  [unwired: 1 in, 1 out]
                }
                event "QUIT": Value Change {
                  # "set flag to stop acquisition loop"
                  n142 = event-data() -> ()  [unwired: 1 in, 6 out]
                  n143 = call <instrlib>:"FGV-B-Scan Active.vi"("Action"=FGV_-_B-Scan_Active_-_Action_[Enum]."B-Scan Finished") -> ("B-Scan In Progress?"=w249:bool)  [unwired: 8 in, 2 out]
                  n144 = local write "B-Scan In Progress?"(w249) -> ()
                  "Stop" <- TRUE ("Stop")
                }
              }
            }
            n145 = while {
              stop <- w72 stop-if-true
              # "Timed scan trigger loop\n(Simple for example code purposes)"
              n146 = local read "Scan Timer Enabled?"() -> (w73:bool)
              n147 = case shown="True" w73 {
                frame False {
                  # "Add a wait so the loop doesn't hog the processor"
                  n148 = Wait (ms)(milliseconds to wait=u32 100) -> ()  [unwired: 1 out]
                }
                frame True {
                  n149 = call <instrlib>:"FGV-B-Scan Active.vi"("Action"=FGV_-_B-Scan_Active_-_Action_[Enum]."Read") -> ("error out"=w76:errorcluster, "B-Scan In Progress?"=w77:bool)  [unwired: 8 in, 1 out]
                  n150 = case shown="True" w77 {
                    tunnel: w76 -> [_ w80]
                    frame False {
                      # "Reset the scan timer flag when B-Scan finishes"
                      n151 = local write "Scan Timer Enabled?"(FALSE ("Scan Timer Enabled?")) -> ()
                    }
                    frame True {
                      # "trigger a CAL 0 when time elapsed"
                      n152 = Unbundle By Name("Timed Scan definition") -> ("Update Rate"=w82:i32)
                      n153 = Wait Until Next ms Multiple(millisecond multiple=w82) -> (millisecond timer value=w81:u32)
                      n154 = flat-sequence {
                        tunnel: w81 -> [_]
                        tunnel: w80 -> [w84]
                        frame #0 {
                          n155 = call <instrlib>:"Start 1 Test Cycle [CAL].vi"("error in (no error)"=w84) -> ()  [unwired: 9 in, 2 out]
                        }
                      }
                    }
                  }
                }
              }
              n156 = flat-sequence {
                tunnel: [w74] -> w72
                frame #0 {
                  n157 = local read "Stop"() -> (w74:bool)
                }
              }
            }
            n158 = control-ref of="A-Scan + Peaks"() -> (w71:refnum<vi>)
            n159 = property on="B-Scan Chart" class="IntGraph (strict)"() -> ("Plot Area Size"=w69:T47)  [unwired: 2 in, 2 out]
            n160 = while {
              tunnel: w71 -> [w89]
              tunnel: [w88] -> w66
              tunnel: w69 -> [w86]
              tunnel: [w85] -> w68
              stop <- w87 stop-if-true
              # "Asynchronous Read from Micropulse"
              n161 = call <instrlib>:"Read MP Message.vi"() -> ("error out"=w90:errorcluster, "scan data info"=w91:T48, "Instrument Message"=w94:string)  [unwired: 7 in, 2 out]
              n162 = call <instrlib>:"Instrument Message History.vi"("Instrument Message"=w94) -> ("Message Count"=→"message count":i32, "Message History out"=→"System Messages":string)  [unwired: 9 in]
              n163 = Unbundle By Name(w91) -> ("Test No."=w92:u32)
              n164 = case shown="1" w92 {
                selector: w92 -> [_ w109]
                tunnel: w91 -> [_ w106]
                tunnel: w90 -> [w97 w111]
                tunnel: w89 -> [_ w108]
                tunnel: [w97 w110] -> w88
                tunnel: w86 -> [_ w99]
                tunnel: [_ w98] -> w85
                frame -1, Default {
                }
                frame 1 {
                  # "To save CPU time and allow for updates due to cursor moves, we restrict unnecessary updates from the uPulse to live data."
                  n165 = local read "Axis No."() -> (w104:u8)
                  n166 = call <instrlib>:"AScan+Peaks to XY Chart.vi"("error in (no error)"=w111, "scan data info"=w106, "Test No."=w109) -> ("error out"=w112:errorcluster, "Echo Range (us)"=w107:dbl, "AScan+Peaks"=w115:cluster{"timebase":dbl[], "data":u16[]}[], "Update Indicators?"=w102:bool, "Running Average PRF"=→"running average PRF":dbl)  [unwired: 3 in, 1 out]
                  n167 = case shown="\"Absolute Scan [FLX+FLZ]\", Default" "Scan Choice" {
                    tunnel: w106 -> [w134 w139 w145]
                    tunnel: [w128 w135 w142] -> w98
                    tunnel: [w132 w141 w146] -> w101
                    tunnel: [w131 w138 w147] -> _
                    tunnel: w104 -> [w130 w137 _]
                    tunnel: [w129 w136 w143] -> w100
                    frame "Absolute Scan [FLX+FLZ]", Default {
                      n168 = local read "FLZ Scan definition"() -> (w133:T29)
                      n169 = call <instrlib>:"B-Scan (LLC messages) DVR.vi"("Scan definition"=w133, "Axis No."=w130, "scan data info"=w134) -> ("Update Display?"=w129:bool, "B-Scan In Progress?"=w132:bool, "B-Scan index"=w131:i32, "data value reference"=w128:refnum<data-value>)  [unwired: 5 in]
                    }
                    frame "Relative Scan [FLR] " {
                      n170 = local read "FLR Scan definition"() -> (w140:T31)
                      n171 = call <instrlib>:"B-Scan (Relative [FLR]) DVR.vi"("Scan definition"=w140, "Axis No."=w137, "scan data info"=w139) -> ("Update Display?"=w136:bool, "B-Scan In Progress?"=w141:bool, "B-Scan index"=w138:i32, "data value reference"=w135:refnum<data-value>)  [unwired: 5 in]
                    }
                    frame "Timed Scan" {
                      n172 = local read "Timed Scan definition"() -> (w144:T33)
                      n173 = call <instrlib>:"B-Scan (Timed) DVR.vi"("Scan definition"=w144, "scan data info"=w145) -> ("Update Display?"=w143:bool, "B-Scan In Progress?"=w146:bool, "B-Scan Index"=w147:i32, "data value reference"=w142:refnum<data-value>)  [unwired: 6 in]
                    }
                  }
                  "B-Scan In Progress?" <- w101
                  n174 = Index Array(array=w115, index="Gate No.") -> (element=→"peak data":cluster{"timebase":dbl[], "data":u16[]})
                  n175 = case shown="True" w102 {
                    tunnel: w115 -> [_ w123]
                    tunnel: w112 -> [w116 w121]
                    tunnel: [w116 w120] -> w110
                    tunnel: w109 -> [_ w119]
                    tunnel: w108 -> [_ w118]
                    tunnel: w107 -> [_ w117]
                    frame False {
                    }
                    frame True {
                      n176 = call <instrlib>:"Adjust Peak Offsets On XY Chart.vi"("error in (no error)"=w121, "Echo Range in"=w117, "AScan+Peaks in"=w123) -> ("error out"=w122:errorcluster, "AScan+Peaks out"=→"A-Scan + Peaks":cluster{"timebase":dbl[], "data":u16[]}[])  [unwired: 7 in]
                      n177 = call <instrlib>:"Draw Gates On XY Chart.vi"("error in (no error)"=w122, "Echo Range"=w117, "XYGraph in"=w118, "Test No."=w119) -> ("error out"=w120:errorcluster)  [unwired: 7 in]
                    }
                  }
                  "live error out" <- w110
                  n178 = case shown="True" w100 {
                    tunnel: w98 -> [_ w126]
                    tunnel: w99 -> [_ w125]
                    frame False {
                    }
                    frame True {
                      n179 = call <instrlib>:"Decimate Data For 2D Intensity Chart - DVR.vi"("Plot Area"=w125, "data value reference"=w126) -> ("Decimated Display"=→"B-Scan Chart":u16[][])  [unwired: 9 in]
                    }
                  }
                }
              }
              n180 = flat-sequence {
                tunnel: [w96] -> w87
                tunnel: w88 -> [_]
                frame #0 {
                  n181 = local read "Stop"() -> (w96:bool)
                }
              }
            }
            n182 = Delete Data Value Reference(data value reference=w68, error in=w66) -> (error out=w67:errorcluster)  [unwired: 1 out]
          }
          frame Error {
          }
        }
        n183 = Select(t=Main_Program_State_-_Enum."Reset HW", s=w61, f=Main_Program_State_-_Enum."Shutdown") -> (s? t:f=w60:T38)
      }
      frame "Reset HW" {
        # "Close the connection to allow for reopening in the \"Init HW\" case"
        n184 = call <instrlib>:"Close.vi"("error in (no error)"=w256) -> ("error out"=w255:errorcluster)  [unwired: 9 in, 1 out]
      }
      frame "Shutdown" {
        # "Terminate the TCP/IP connection"
        n185 = local write "Stop"(FALSE ("stop")) -> ()
        n186 = call <instrlib>:"Close.vi"() -> ()  [unwired: 10 in, 2 out]
      }
    }
  }
